vi "InitializeDotsByIndex.vi"(8 "error in (no error)":errorcluster, 10 "Dots":string[](array[string]), 11 "Setting Database in":refnum<class "Setting Database.lvclass">) -> (0 "error out":errorcluster, 3 "Setting Database out":refnum<class "Setting Database.lvclass">)   [LabVIEW 2019, in "Setting Database.lvclass"]
uses:
  Setting Database.lvclass
  Setting Database.lvclass/Setting Database.ctl
  <vilib>/Utility/sysdir.llb/Get System Directory.vi
  Dot Settings/Dot Settings.lvclass
  C:/Users/Albro/Documents/GitHub/AFM-Lithography/lvsrc/Classes/Settings/ObjectSettings/ObjectSettings.lvclass
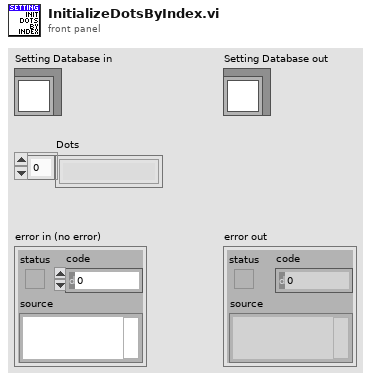
[diagram p1: front panel]
types:
  T1 = cluster{"Path":i32, "Funnel":i32, "Rectangle":i32, "Dot":i32}
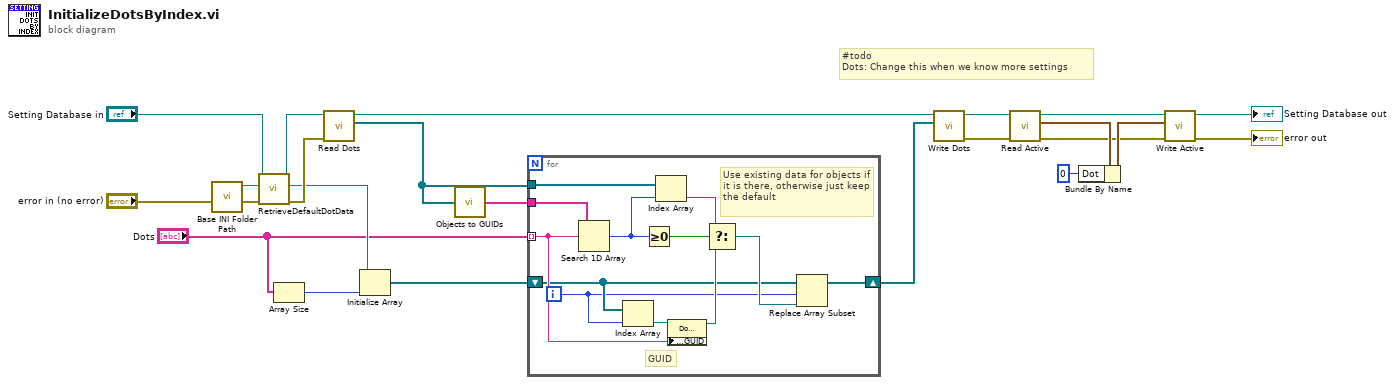
[diagram p0: block diagram]
diagram:
  # "#todo\nDots: Change this when we know more settings"
  n1 = call "Base INI Folder Path.vi"() -> ("Base Path"=w10:path)  [unwired: 11 in]
  n2 = call "RetrieveDefaultDotData.vi"("error in (no error)"="error in (no error)", "Path"=w10, "Setting Database In"="Setting Database in") -> ("error out"=w12:errorcluster, "Dot Settings out"=w7:refnum<class "Dot Settings.lvclass">, "Setting Database Out"=w8:refnum<class "Setting Database.lvclass">)  [unwired: 6 in]
  n3 = Array Size(array="Dots") -> (size(s)=w6:i32)
  n4 = call "Read Dots.vi"("error in (no error)"=w12, "Setting Database in"=w8) -> ("Dots"=w5:refnum<class "Dot Settings.lvclass">[], "Setting Database out"=w13:refnum<class "Setting Database.lvclass">)  [unwired: 7 in, 1 out]
  n5 = Initialize Array(w7, w6) -> (w2:refnum<class "Dot Settings.lvclass">[])
  n6 = call "Objects to GUIDs.vi"("Objects"=w5) -> ("GUIDs"=w4:string[])  [unwired: 3 in, 1 out]
  n7 = for {
    tunnel: w5 -> [w32]
    shift-right: [w34] -> w1
    shift-left: w2 -> [w24]
    tunnel: w4 -> [w31]
    tunnel: "Dots" -> [w29] mode=indexing
    i -> [w23]
    # "GUID"
    # "Use existing data for objects if it is there, otherwise just keep the default"
    n8 = Search 1D Array(1D array=w31, element=w29) -> (index of element=w33:i32)  [unwired: 1 in]
    n9 = Index Array(array=w24, index=w23) -> (element=w30:refnum<class "Dot Settings.lvclass">)
    n10 = Greater Or Equal To 0?(x=w33) -> (x >= 0?=w28:bool)
    n11 = Index Array(array=w32, index=w33) -> (element=w27:refnum<class "Dot Settings.lvclass">)
    n12 = property class="Dot Settings.lvclass"(reference=w30, "Accessors:GUID"=w29) -> (reference out=w25:refnum<class "Dot Settings.lvclass">)  [unwired: 1 in, 1 out]
    n13 = Select(t=w27, s=w28, f=w25) -> (s? t:f=w26:refnum<class "Dot Settings.lvclass">)
    n14 = Replace Array Subset(array=w24, new element=w26, index=w23) -> (w34:refnum<class "Dot Settings.lvclass">[])
  }
  n15 = call "Write Dots.vi"("Dots"=w1, "Setting Database in"=w13) -> ("error out"=w15:errorcluster, "Setting Database out"=w21:refnum<class "Setting Database.lvclass">)  [unwired: 8 in]
  n16 = call "Read Active.vi"("error in (no error)"=w15, "Setting Database in"=w21) -> ("error out"=w16:errorcluster, "Active"=w19:T1, "Setting Database out"=w22:refnum<class "Setting Database.lvclass">)  [unwired: 7 in]
  n17 = Bundle By Name(cluster=w19, "Dot"=0) -> (w18:T1)
  n18 = call "Write Active.vi"("error in (no error)"=w16, "Active"=w18, "Setting Database in"=w22) -> ("error out"=→"error out":errorcluster, "Setting Database out"=→"Setting Database out":refnum<class "Setting Database.lvclass">)  [unwired: 7 in]
